vi "DDS Set Single-Tone Profile.vi"(0 "DDS ref in":T2={"NI USB-8451 device reference"="", "DIO port"=0, "Serial Clock Rate [kHz]"=1000}, 1 "Amplitude [dBm] (0)":dbl, 2 "Phase Offset [rad] (0)":dbl, 3 "Frequency [MHz] (0)":dbl, 5 "Channel Parameters":T1, 7 "Profile (0)":u8, 11 "error in (no error)":errorcluster, 12 "channel number (1)":u8=1 min=1 max=4 step=1) -> (4 "DDS ref out":T2={"NI USB-8451 device reference"="", "DIO port"=0, "Serial Clock Rate [kHz]"=1000}, 6 "Write Data":u8[](array[numeric]), 15 "error out":errorcluster)   [LabVIEW 2013, in "DDS.lvlib"]
doc: "Sets the amplitude/phase/frequency of the given single-tone profile on the specified channel.\n\nThe amplitude is given in units of dBm and is converted to a 14-bit amplitude scale factor using the channel's full scale output power as a parameter. The phase is given in radians and is converted to a 16-bit phase offset word. The frequency is given in MHz and is converted to a 32-bit frequency tuning word using the channel's reference clock rate as a parameter."
uses:
  DDS.lvlib
  Controls/DDS Box Device Reference.ctl
  <vilib>/ni845x/ni845x.llb/ni845xControl.ctl
  Controls/AD9910 registers.ctl
panel:
  out "Phase Offset Word":u32 format="%04x"
  out "Frequency Tuning Word":u32 format="%08x"
  out "Amplitude Scale Factor":u32 format="%04x"
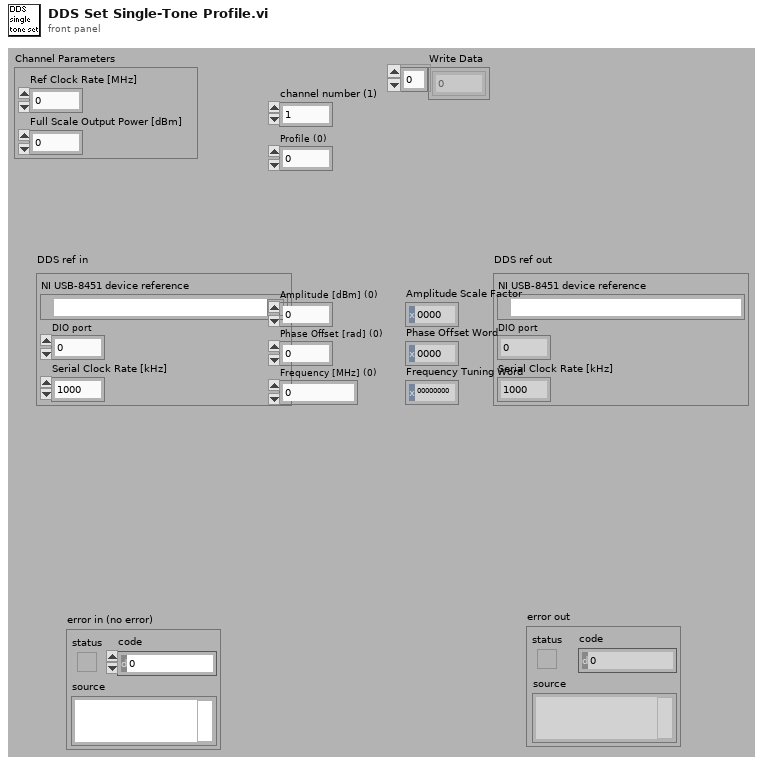
[diagram p1: front panel]
types:
  T1 = cluster{"Ref Clock Rate [MHz]":dbl, "Full Scale Output Power [dBm]":dbl}
  T2 = typedef "DDS.lvlib/DDS Box Device Reference.ctl" = cluster{"NI USB-8451 device reference":T3, "DIO port":u8, "Serial Clock Rate [kHz]":u16}
  T3 = typedef "ni845xControl.ctl" = refnum<k21>
  T4 = typedef "DDS.lvlib/AD9910 registers.ctl" = enum16{"CFR1", "CFR2", "CFR3", "Auxiliary DAC Control", "I/0 Update Rate", "Frequency Tuning Word", "Phase Offset Word", "Amplitude Scale Factor", "Multichip Sync", "Digital Ramp Limit", "Digital Ramp Step Size", "Digital Ramp Rate", "Single Tone Profile 0", "Single Tone Profile 1", "Single Tone Profile 2", "Single Tone Profile 3", "Single Tone Profile 4", "Single Tone Profile 5", "Single Tone Profile 6", "Single Tone Profile 7", "RAM Profile 0", "RAM Profile 1", "RAM Profile 2", "RAM Profile 3", "RAM Profile 4", "RAM Profile 5", "RAM Profile 6", "RAM Profile 7", "RAM"}
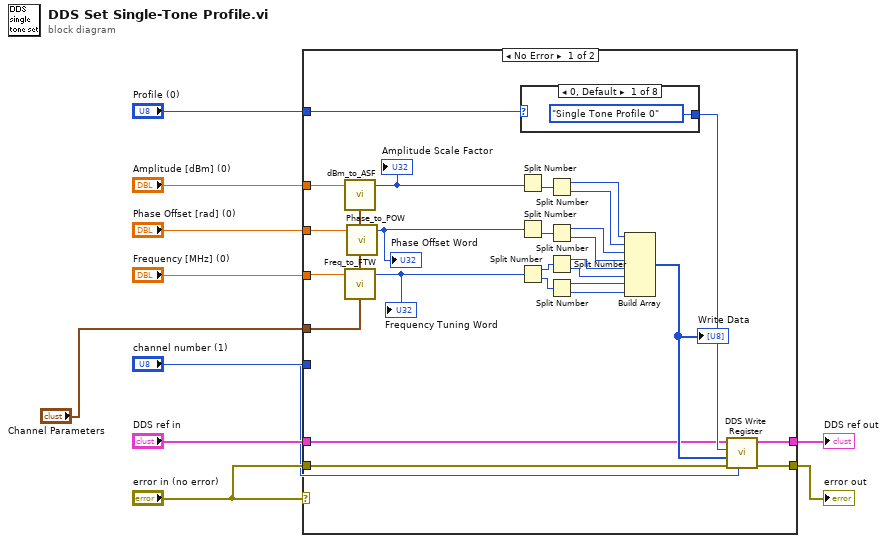
[diagram p0: block diagram]
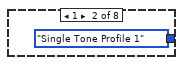
[diagram p2: hidden frame]
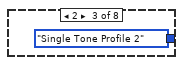
[diagram p3: hidden frame]
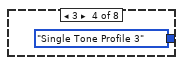
[diagram p4: hidden frame]
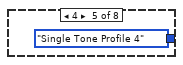
[diagram p5: hidden frame]
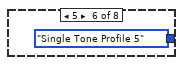
[diagram p6: hidden frame]
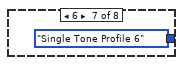
[diagram p7: hidden frame]
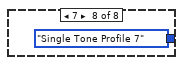
[diagram p8: hidden frame]
diagram:
  n1 = case shown="No Error" "error in (no error)" {
    tunnel: "error in (no error)" -> [w21 w47]
    tunnel: [w23 w47] -> w5
    tunnel: "Amplitude [dBm] (0)" -> [w15 _]
    tunnel: "Phase Offset [rad] (0)" -> [w17 _]
    tunnel: "Profile (0)" -> [w20 _]
    tunnel: "DDS ref in" -> [w19 w46]
    tunnel: [w22 w46] -> w4
    tunnel: "Frequency [MHz] (0)" -> [w12 _]
    tunnel: "channel number (1)" -> [w18 _]
    tunnel: "Channel Parameters" -> [w13 _]
    frame No Error {
      n2 = call "dBm_to_ASF.vi"("Amplitude (dBm)"=w15, "Channel Parameters"=w13) -> ("ASF"=w14:u32)  [unwired: 25 in]
      "Amplitude Scale Factor" <- w14
      n3 = call "Freq_to_FTW.vi"("Frequency (MHz)"=w12, "Channel Parameters"=w13) -> ("FTW (32bit)"=w11:u32)  [unwired: 25 in]
      "Frequency Tuning Word" <- w11
      n4 = call "Phase_to_POW.vi"("Phase (rad.)"=w17) -> ("POW"=w16:u32)  [unwired: 26 in]
      "Phase Offset Word" <- w16
      n5 = Split Number(x=w14) -> (lo(x)=w34:u16)  [unwired: 1 out]
      n6 = Split Number(x=w16) -> (lo(x)=w35:u16)  [unwired: 1 out]
      n7 = Split Number(x=w11) -> (hi(x)=w36:u16, lo(x)=w37:u16)
      n8 = case shown="0, Default" w20 {
        tunnel: [AD9910_registers."Single Tone Profile 0" ("Register") AD9910_registers."Single Tone Profile 1" ("Register") AD9910_registers."Single Tone Profile 2" ("Register") AD9910_registers."Single Tone Profile 3" ("Register") AD9910_registers."Single Tone Profile 4" ("Register") AD9910_registers."Single Tone Profile 5" ("Register") AD9910_registers."Single Tone Profile 6" ("Register") AD9910_registers."Single Tone Profile 7" ("Register")] -> w24
        frame 0, Default {
        }
        frame 1 {
        }
        frame 2 {
        }
        frame 3 {
        }
        frame 4 {
        }
        frame 5 {
        }
        frame 6 {
        }
        frame 7 {
        }
      }
      n9 = Split Number(x=w34) -> (hi(x)=w26:u8, lo(x)=w27:u8)
      n10 = Split Number(x=w35) -> (hi(x)=w28:u8, lo(x)=w29:u8)
      n11 = Split Number(x=w36) -> (hi(x)=w30:u8, lo(x)=w31:u8)
      n12 = Split Number(x=w37) -> (hi(x)=w32:u8, lo(x)=w33:u8)
      n13 = Build Array(w26, w27, w28, w29, w30, w31, w32, w33) -> (w25:u8[])
      "Write Data" <- w25
      n14 = call "DDS Write Register.vi"("channel number (1)"=w18, "error in (no error)"=w21, "Write Data"=w25, "Register"=w24, "DDS ref in"=w19) -> ("error out"=w23:errorcluster, "DDS ref out"=w22:T2)  [unwired: 4 in, 1 out]
    }
    frame Error {
    }
  }
  "error out" <- w5
  "DDS ref out" <- w4
